vi "SRV_Sensor View Tab_Initialize Captions.vi"(5 "Sensor View refs":T1, 11 "error in (no error)":errorcluster) -> (6 "Sensor View refs dup":T1, 15 "error out":errorcluster)   [LabVIEW 2009]
uses:
  SRV_Sensor View refs.ctl
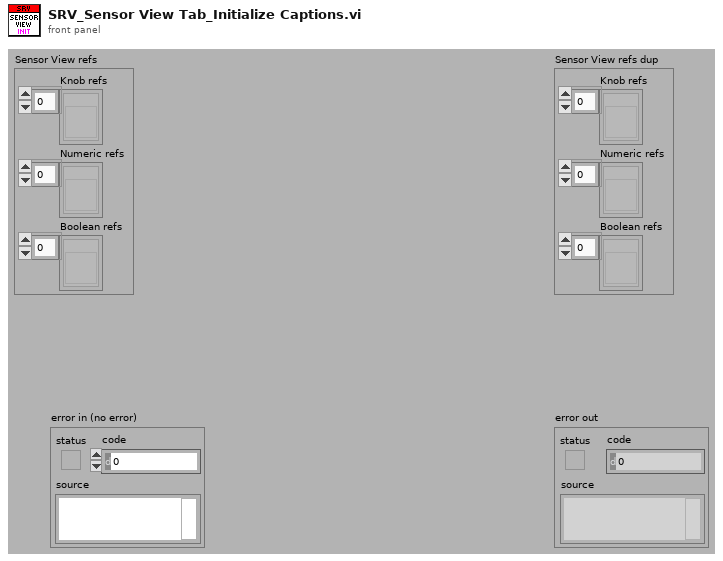
[diagram p1: front panel]
types:
  T1 = typedef "SRV_Sensor View refs.ctl" = cluster{"Knob refs":refnum<vi>[], "Numeric refs":refnum<vi>[], "Boolean refs":refnum<vi>[]}
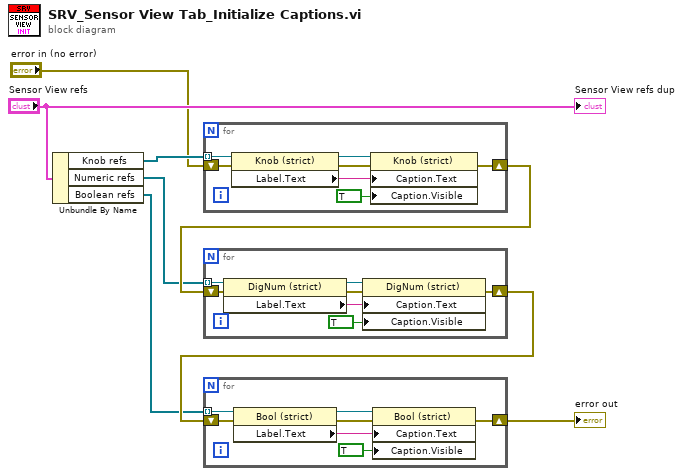
[diagram p0: block diagram]
diagram:
  n1 = Unbundle By Name("Sensor View refs") -> ("Knob refs"=w8:refnum<vi>[], "Numeric refs"=w5:refnum<vi>[], "Boolean refs"=w4:refnum<vi>[])
  n2 = for {
    tunnel: w8 -> [w15] mode=indexing
    shift-right: [w10] -> w7
    shift-left: "error in (no error)" -> [w11]
    n3 = property class="Knob (strict)"(reference=w15, error in=w11) -> (reference out=w14:refnum<vi>, error out=w13:errorcluster, "Label.Text"=w12:string)
    n4 = property class="Knob (strict)"(reference=w14, error in=w13, "Caption.Text"=w12, "Caption.Visible"=TRUE) -> (error out=w10:errorcluster)  [unwired: 1 out]
  }
  n5 = for {
    tunnel: w5 -> [w22] mode=indexing
    shift-right: [w17] -> w6
    shift-left: w7 -> [w18]
    n6 = property class="DigNum (strict)"(reference=w22, error in=w18) -> (reference out=w21:refnum<vi>, error out=w20:errorcluster, "Label.Text"=w19:string)
    n7 = property class="DigNum (strict)"(reference=w21, error in=w20, "Caption.Text"=w19, "Caption.Visible"=TRUE) -> (error out=w17:errorcluster)  [unwired: 1 out]
  }
  n8 = for {
    tunnel: w4 -> [w29] mode=indexing
    shift-right: [w24] -> w3
    shift-left: w6 -> [w25]
    n9 = property class="Bool (strict)"(reference=w29, error in=w25) -> (reference out=w28:refnum<vi>, error out=w27:errorcluster, "Label.Text"=w26:string)
    n10 = property class="Bool (strict)"(reference=w28, error in=w27, "Caption.Text"=w26, "Caption.Visible"=TRUE) -> (error out=w24:errorcluster)  [unwired: 1 out]
  }
  "error out" <- w3
  "Sensor View refs dup" <- "Sensor View refs"
